vi "ProdaNG.Example.GetProductComponent.vi"() -> ()   [LabVIEW 2016]
uses:
  Controls/ProdaNG.ProductComponent.ctl
panel:
  out "ProdComponents":T1[](array[typedef])
  in  "serialNumber 1":string="30010025161214"
  out "error out":errorcluster
  in  "error in (no error)":errorcluster
  in  "wabcoNumber 1":string="4430203001"
  out "DataBase time":string
  in  "Connection string":string="lcptb/lcptb@PRODA_WPK"
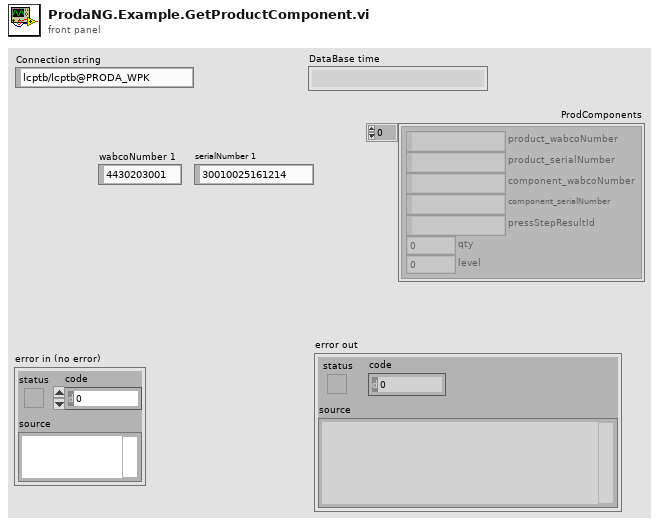
[diagram p1: front panel]
types:
  T1 = typedef "ProdaNG.ProductComponent.ctl" = cluster{"product_wabcoNumber":string, "product_serialNumber":string, "component_wabcoNumber":string, "component_serialNumber":string, "pressStepResultId":string, "qty":i32, "level":i32}
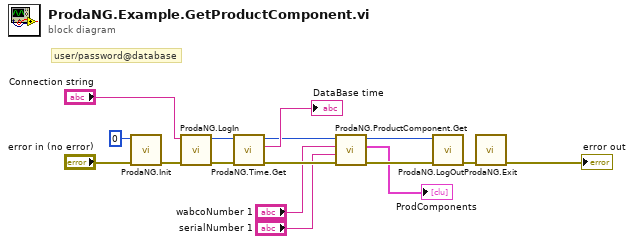
[diagram p0: block diagram]
diagram:
  # "user/password@database"
  n1 = call "ProdaNG.Init.vi"("error in (no error)"="error in (no error)", "numContexts (0: unlimited)"=0 ("numContexts")) -> ("error out"=w15:errorcluster)  [unwired: 9 in]
  n2 = call "ProdaNG.LogIn.vi"("error in"=w15, "ConnectionString"="Connection string") -> ("error out"=w11:errorcluster, "dbHandle"=w12:i32)  [unwired: 7 in, 1 out]
  n3 = call "ProdaNG.Time.Get.vi"("error in"=w11, "dbHandleIn"=w12) -> ("error out"=w7:errorcluster, "timeStr"=→"DataBase time":string, "dbHandle"=w6:i32)  [unwired: 5 in, 1 out]
  n4 = call "ProdaNG.ProductComponent.Get.vi"("error in (no error)"=w7, "serialNumber"="serialNumber 1", "wabcoNumber"="wabcoNumber 1", "dbHandle"=w6) -> ("error out"=w5:errorcluster, "ProdComponents"=→"ProdComponents":T1[], "dbHandle out"=w4:i32)  [unwired: 5 in]
  n5 = call "ProdaNG.LogOut.vi"("error in"=w5, "dbHandleIn"=w4) -> ("error out"=w16:errorcluster)  [unwired: 9 in]
  n6 = call "ProdaNG.Exit.vi"("error in (no error)"=w16) -> ("error out"=→"error out":errorcluster)  [unwired: 10 in]
